vi "Calculator.vi"() -> ()   [LabVIEW 2015]
panel:
  in  "Numeric 2":dbl
  in  "Numeric":dbl
  in  "stop":bool
  in  "Boolean 2":bool
  in  "Boolean 1":bool
  # "+\n*              /\n       -"
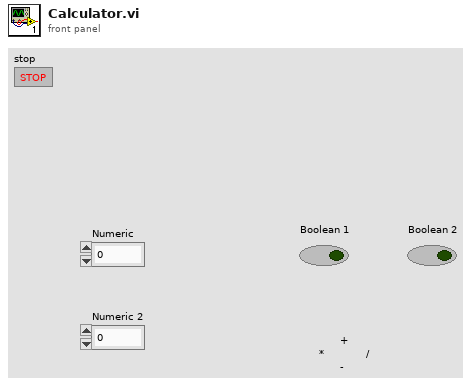
[diagram p1: front panel]
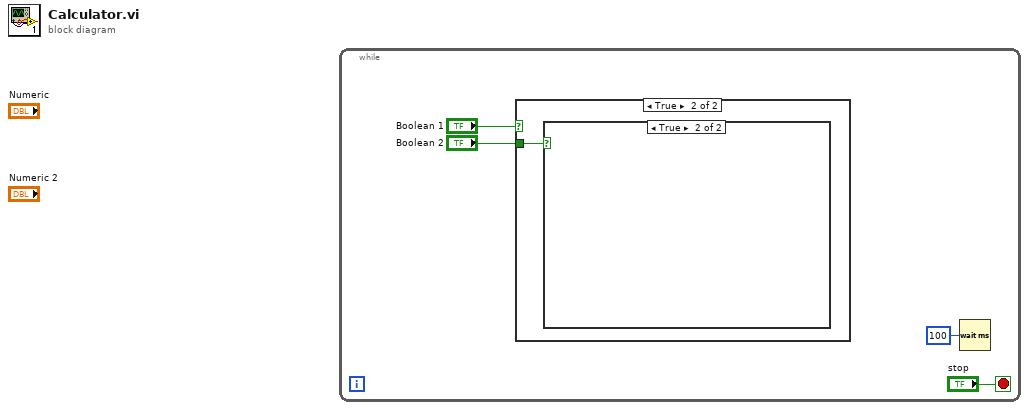
[diagram p0: block diagram]
diagram:
  n1 = while {
    stop <- "stop" stop-if-true
    n2 = case shown="True" "Boolean 1" {
      tunnel: "Boolean 2" -> [w5 w6]
      frame False {
        n3 = case shown="True" w5 {
          frame False {
          }
          frame True {
          }
        }
      }
      frame True {
        n4 = case shown="True" w6 {
          frame False {
          }
          frame True {
          }
        }
      }
    }
    n5 = Wait (ms)(milliseconds to wait=u32 100) -> ()  [unwired: 1 out]
  }
